vi "UserEventUnderstanding.vi"() -> ()   [LabVIEW 2019]
panel:
  out "all upper case string":string
  in  "Enter your name":string
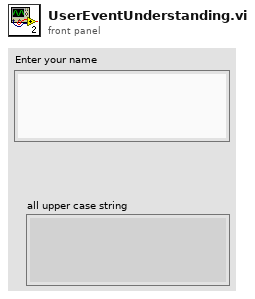
[diagram p1: front panel]
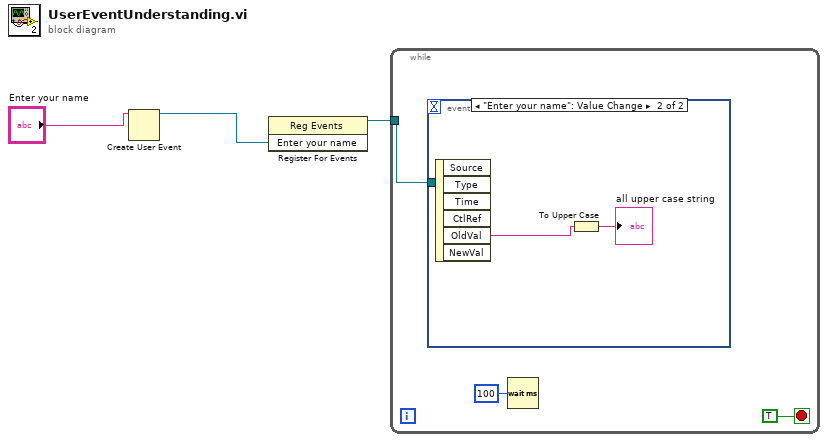
[diagram p0: block diagram]
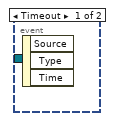
[diagram p2: hidden frame]
diagram:
  n1 = Create User Event(user event datatype="Enter your name") -> (user event=w2:refnum<user-event>)  [unwired: 1 in, 1 out]
  n2 = register-events(w2) -> (reference out=w1:refnum<event-registration>)  [unwired: 2 in, 1 out]
  n3 = while {
    tunnel: w1 -> [w4]
    stop <- TRUE stop-if-true
    n4 = event shown="[1] \"Enter your name\": Value Change" {
      selector: _ -> [_ _]
      dyn-events: _ -> [_ _]
      timeout: _ -> [_ _]
      tunnel: w4 -> [_ _]
      event Timeout {
        n5 = event-data() -> ()  [unwired: 1 in, 3 out]
      }
      event "Enter your name": Value Change {
        n6 = event-data() -> ("OldVal"=w8:string)  [unwired: 1 in, 5 out]
        n7 = To Upper Case(1:w8) -> (0:→"all upper case string":string)
      }
    }
    n8 = Wait (ms)(milliseconds to wait=u32 100) -> ()  [unwired: 1 out]
  }
